vi "Add Frames.vi"(8 "error in (no error)":errorcluster, 11 "Node Ptr":u64 format="%.0x") -> ()   [LabVIEW 2020, in "FlexRay Custom Device System Explorer.lvlib"]
uses:
  FlexRay Custom Device System Explorer.lvlib
  Shared/FRConfig.ctl
  Shared/FRInterface.ctl
  <vilib>/Utility/error.llb/DialogType.ctl
  Shared/AddFramesState.ctl
  Shared/FRFrameType.ctl
  <vilib>/NI VeriStand/Custom Device API/Custom Device Channel Type.ctl
  <vilib>/NI VeriStand/Custom Device API/Custom Device Item Ref.ctl
  <vilib>/NI VeriStand/Custom Device API/Custom Device Channel.ctl
  Shared/Constants.vi
  <vilib>/NI VeriStand/Custom Device API/Get Item Property (Variant).vi
  Shared/FlexRay Custom Device Shared.lvlib
  <resource>/objmgr/xnet.rc
  <vilib>/NI VeriStand/Custom Device API/Custom Device API.lvlib
panel:
  in  "Add Selection":bool
  in  "Frames":i32[](listbox)
  in  "Reverse":bool
  in  "Cancel":bool
  in  "Add All":bool
  in  "ECU":u16(ring)
  out "error out":errorcluster
  in  "Tag":string
  # "Use ctrl or shift to select multiple frames"
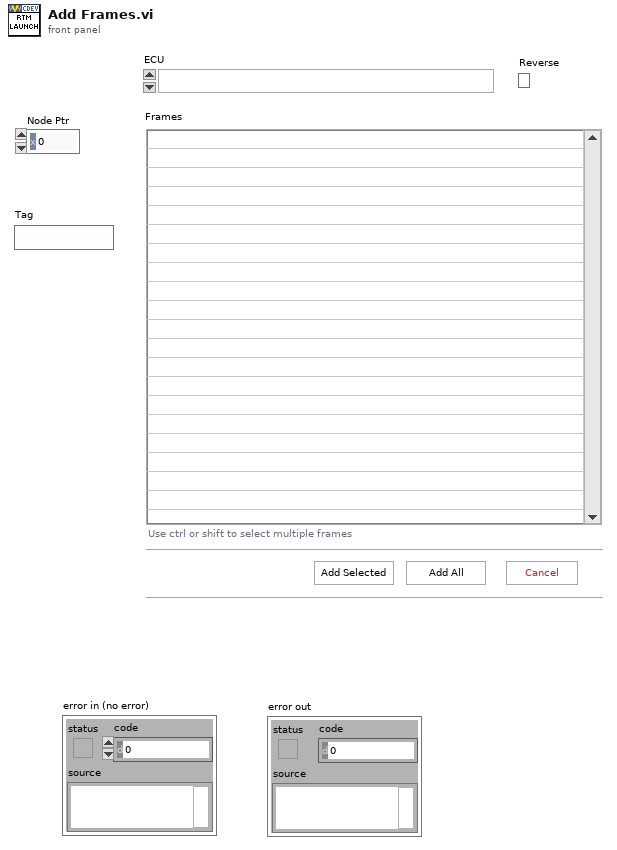
[diagram p1: front panel]
types:
  T1 = typedef "FlexRay Custom Device Shared.lvlib/AddFramesState.ctl" = enum16{"Init", "UserInput", "Action", "Cleanup"}
  T2 = typedef "DialogType.ctl" = u16
  T3 = typedef "FlexRay Custom Device Shared.lvlib/FRConfig.ctl" = cluster{"FlexRay Interface":T4, "XNET Database":refnum<k21>, "XNET Cluster":refnum<k21>, "ColdStart ID":u32, "Termination":bool}
  T4 = typedef "FlexRay Custom Device Shared.lvlib/FRInterface.ctl" = u16
  T5 = typedef "Custom Device API.lvlib/Custom Device Item Info.ctl" = cluster{"Name":string, "Is Channel":bool, "GUID":string, "Is Waveform":bool}
  T6 = typedef "Custom Device API.lvlib/Custom Device Item Ref.ctl" = u64
  T7 = typedef "Custom Device API.lvlib/Custom Device Channel Type.ctl" = enum16{"Input", "Output"}
  T8 = typedef "FlexRay Custom Device Shared.lvlib/FRFrameType.ctl" = u32
  T9 = typedef "Custom Device API.lvlib/Custom Device Channel.ctl" = cluster{"Type":T7, "Units":string, "Default Value":dbl, "Faultable":bool, "Scalable":bool}
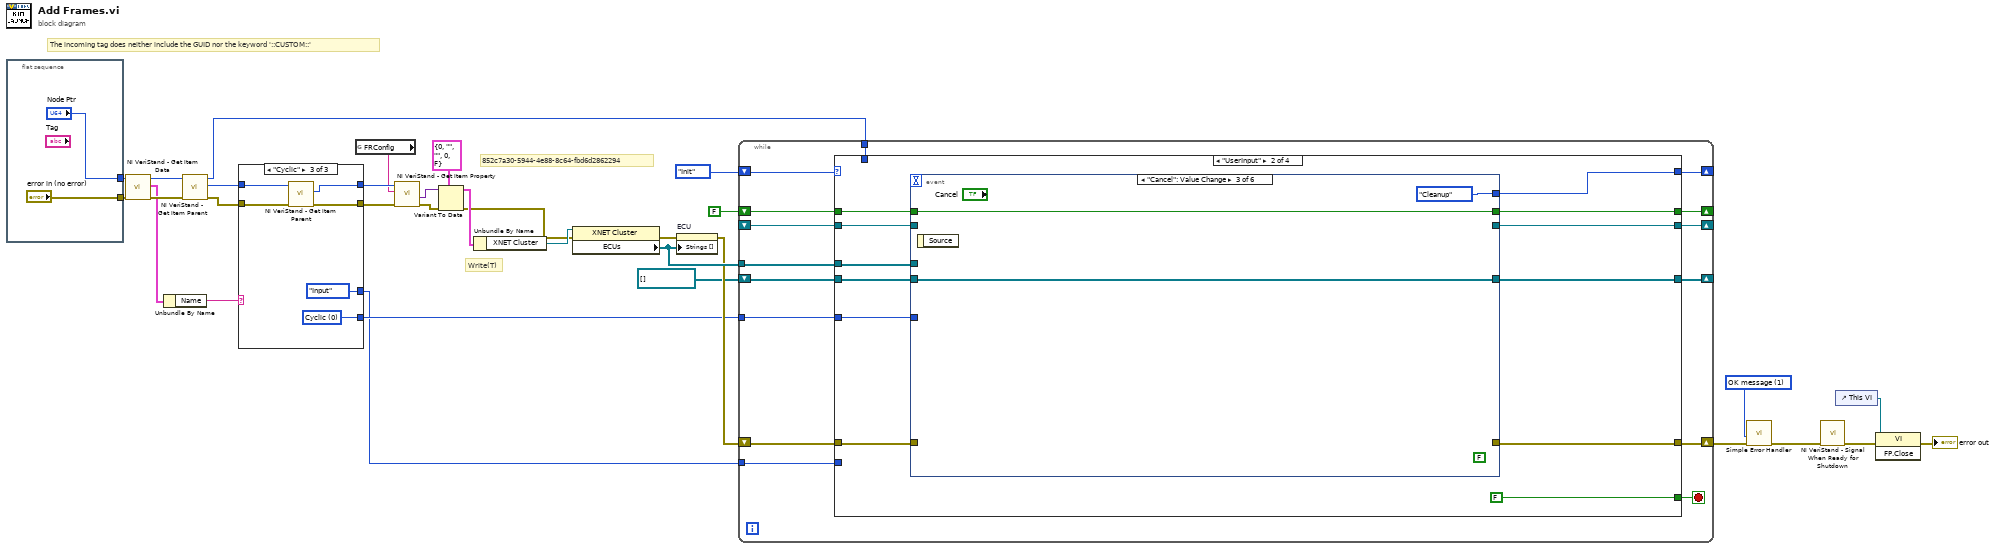
[diagram p0: block diagram]
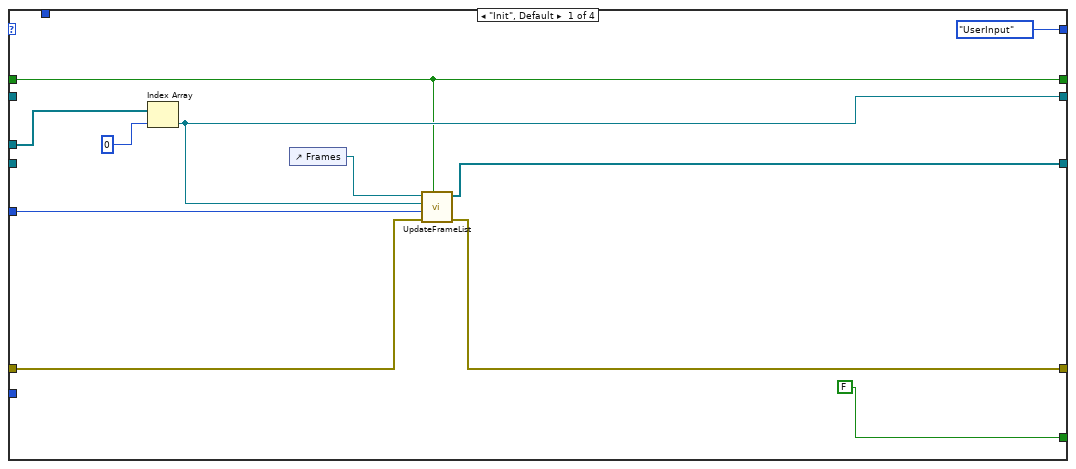
[diagram p2: hidden frame]
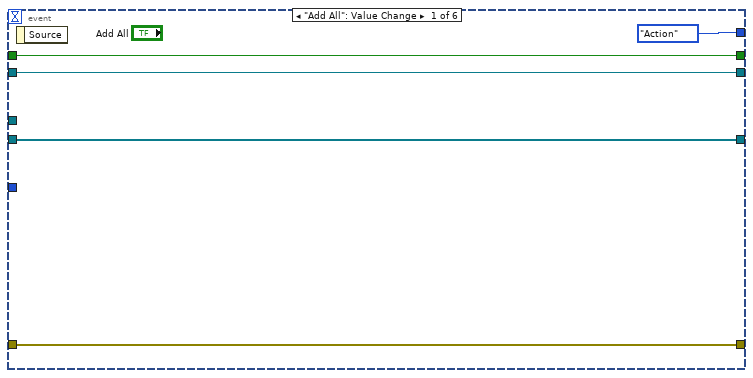
[diagram p3: hidden frame]
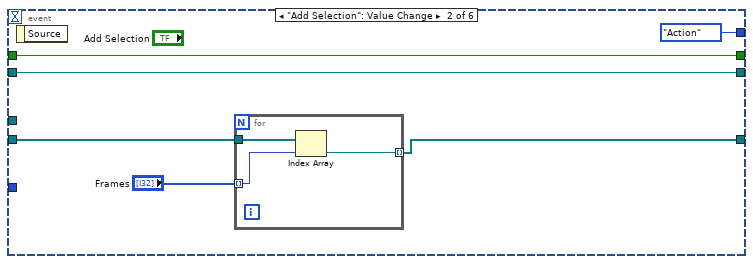
[diagram p4: hidden frame]
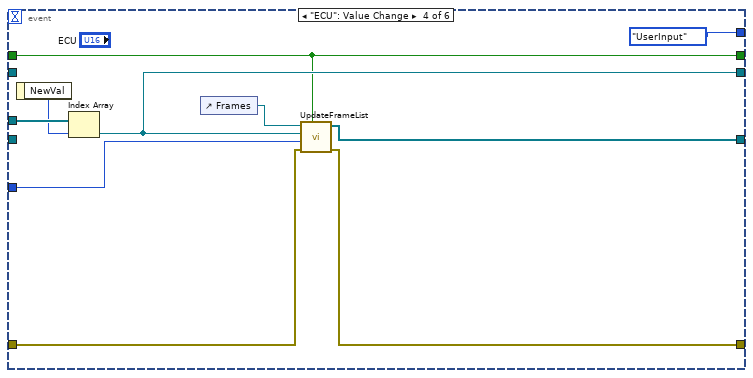
[diagram p5: hidden frame]
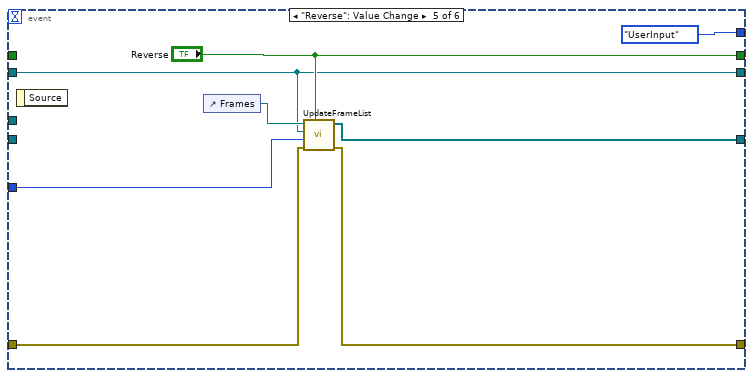
[diagram p6: hidden frame]
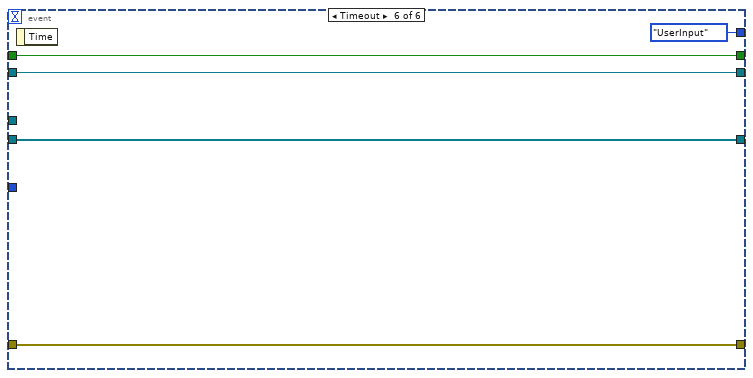
[diagram p7: hidden frame]
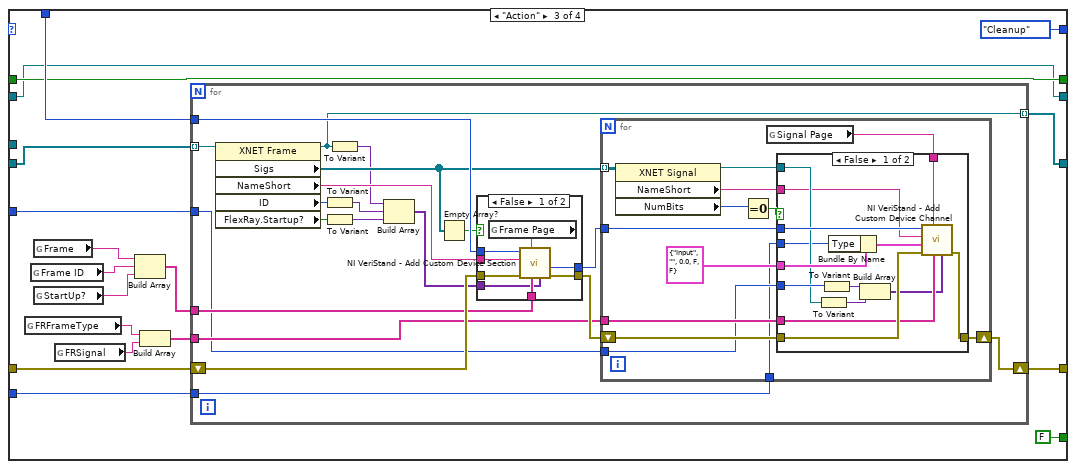
[diagram p8: hidden frame]
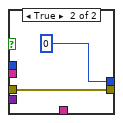
[diagram p9: hidden frame]
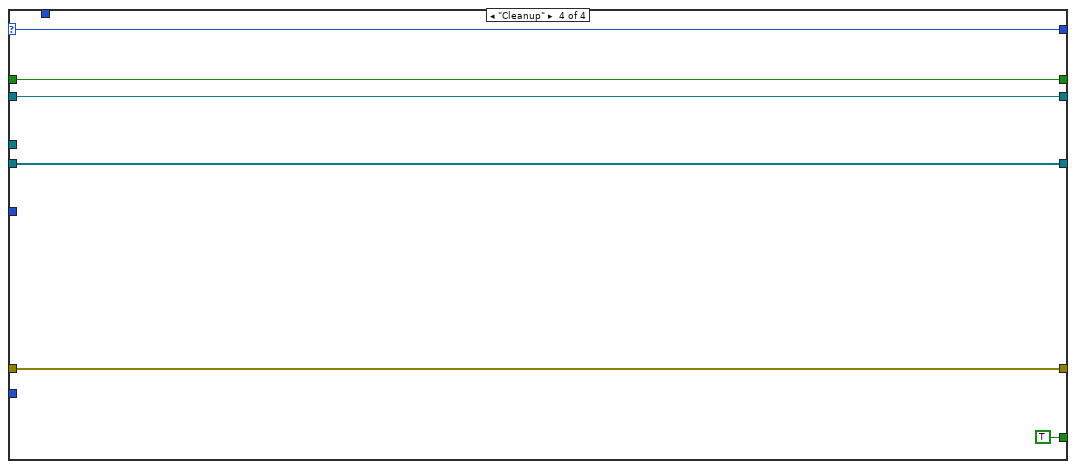
[diagram p11: hidden frame]
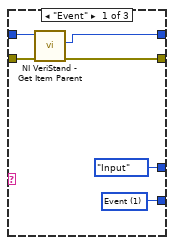
[diagram p12: hidden frame]
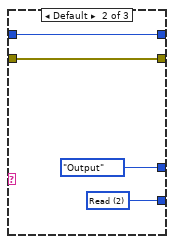
[diagram p13: hidden frame]
diagram:
  w12 = T2 1 items=["no dialog", "OK message", "continue or stop message", "OK message + warnings", "continue/stop + warnings"] ("type of dialog (OK msg:1)")
  # "852c7a30-5944-4e88-8c64-fbd6d2862294"
  # "Write(T)"
  # "The incoming tag does neither include the GUID nor the keyword '::CUSTOM::'"
  n1 = flat-sequence {
    tunnel: ["Node Ptr"] -> w24
    tunnel: ["error in (no error)"] -> w23
    frame #0 {
    }
  }
  n2 = call <vilib>:"NI VeriStand - Get Item Data.vi"("error in (no error)"=w23, "Item Ref in"=w24) -> ("error out"=w22:errorcluster, "Item Info"=w21:T5, "Item Ref out"=w5:T6)  [unwired: 6 in, 1 out]
  n3 = Unbundle By Name(w21) -> ("Name"=w20:string)
  n4 = call <vilib>:"NI VeriStand - Get Item Parent.vi"("error in (no error)"=w22, "Item Ref in"=w5) -> ("error out"=w14:errorcluster, "Parent Ref"=w26:T6, "Item Ref out"=w1:T6)  [unwired: 6 in, 1 out]
  n5 = case shown="\"Cyclic\"" w20 {
    tunnel: [w36 w42 w50] -> w4
    tunnel: w26 -> [w40 w44 w49]
    tunnel: [w39 w44 w48] -> w19
    tunnel: w14 -> [w38 w43 w47]
    tunnel: [w37 w43 w46] -> w25
    tunnel: [Custom_Device_Channel_Type."Input" ("Type") Custom_Device_Channel_Type."Output" ("Type") Custom_Device_Channel_Type."Input" ("Type")] -> w2
    frame "Event" {
      w36 = T8 1 items=["Cyclic", "Event", "Read"] ("FlexRay:Timing Type")
      n6 = call <vilib>:"NI VeriStand - Get Item Parent.vi"("error in (no error)"=w38, "Item Ref in"=w40) -> ("error out"=w37:errorcluster, "Parent Ref"=w39:T6)  [unwired: 6 in, 2 out]
    }
    frame Default {
      w42 = T8 2 items=["Cyclic", "Event", "Read"] ("FlexRay:Timing Type")
    }
    frame "Cyclic" {
      w50 = T8 0 items=["Cyclic", "Event", "Read"] ("FlexRay:Timing Type")
      n7 = call <vilib>:"NI VeriStand - Get Item Parent.vi"("error in (no error)"=w47, "Item Ref in"=w49) -> ("error out"=w46:errorcluster, "Parent Ref"=w48:T6)  [unwired: 6 in, 2 out]
    }
  }
  n8 = global read "Constants.vi" "FRConfig"() -> (w18:string)
  n9 = call-poly <vilib>:"NI VeriStand - Get Item Property.vi"("error in (no error)"=w25, "Property Name"=w18, "Item Ref in"=w19) -> ("error out"=w31:errorcluster, "Value"=w32:variant)  [unwired: 5 in, 2 out]
  n10 = Variant To Data(error in=w31, type=T3 {"FlexRay Interface"=0, "XNET Database"="", "XNET Cluster"="", "ColdStart ID"=0, "Termination"=FALSE} ("FRConfig"), Variant=w32) -> (data=w29:T3, error out=w27:errorcluster)
  n11 = Unbundle By Name(w29) -> ("XNET Cluster"=w28:refnum<k21>)
  n12 = property class="XNET Cluster"(reference=w28, error in=w27) -> (error out=w10:errorcluster, "ECUs"=w11:refnum<k21>[])  [unwired: 1 out]
  n13 = property on="ECU" class="Ring (strict)"(error in=w10, "Strings []"=w11) -> (error out=w9:errorcluster)  [unwired: 1 in, 1 out]
  n14 = while {
    tunnel: w11 -> [w65]
    tunnel: w4 -> [w63]
    shift-right: [w52] -> _
    shift-left: refnum<k21>[] [] -> [w62]
    shift-right: [w53] -> w3
    shift-left: w9 -> [w61]
    shift-right: [w60] -> _
    shift-left: FALSE ("Reverse") -> [w59]
    shift-right: [w55] -> _
    shift-left: AddFramesState."Init" -> [w57]
    shift-right: [w58] -> _
    shift-left: _ -> [w56]
    tunnel: w1 -> [w54]
    tunnel: w2 -> [w51]
    stop <- w64 stop-if-true
    n15 = case shown="\"UserInput\"" w57 {
      selector: w57 -> [_ _ _ w210]
      tunnel: w65 -> [w76 w88 _ _]
      tunnel: [FALSE FALSE FALSE TRUE] -> w64
      tunnel: w63 -> [w72 w87 w130 _]
      tunnel: [w66 w86 w132 w207] -> w52
      tunnel: w62 -> [_ w85 w134 w207]
      tunnel: [w68 w84 w138 w208] -> w53
      tunnel: w61 -> [w70 w83 w133 w208]
      tunnel: [w69 w82 w137 w205] -> w60
      tunnel: w59 -> [w69 w81 w137 w205]
      tunnel: [w71 w80 w136 w206] -> w58
      tunnel: w56 -> [_ w77 w136 w206]
      tunnel: [AddFramesState."UserInput" w79 AddFramesState."Cleanup" w210] -> w55
      tunnel: w54 -> [_ _ w139 _]
      tunnel: w51 -> [_ _ w129 _]
      frame "Init", Default {
        n16 = Index Array(array=w76, index=0) -> (element=w71:refnum<k21>)
        n17 = control-ref of="Frames"() -> (w67:refnum<vi>)
        n18 = call "UpdateFrameList.vi"("Reverse"=w69, "error in (no error)"=w70, "FlexRay:Timing Type"=w72, "XNET ECU"=w71, "ListBox in"=w67) -> ("error out"=w68:errorcluster, "Frames"=w66:refnum<k21>[])  [unwired: 5 in]
      }
      frame "UserInput" {
        n19 = event shown="[2] \"Cancel\": Value Change" {
          selector: _ -> [_ _ _ _ _ _]
          dyn-events: _ -> [_ _ _ _ _ _]
          timeout: _ -> [_ _ _ _ _ _]
          tunnel: w88 -> [_ _ _ w115 _ _]
          tunnel: w87 -> [_ _ _ w110 w119 _]
          tunnel: [w91 w94 w105 w107 w118 w127] -> w86
          tunnel: w85 -> [w91 w95 w105 _ _ w127]
          tunnel: [w89 _ _ w108 w117 w128] -> w84
          tunnel: w83 -> [w89 _ _ w109 w116 w128]
          tunnel: [w93 w98 w104 w111 "Reverse" w126] -> w82
          tunnel: w81 -> [w93 w98 w104 w111 _ w126]
          tunnel: [w90 w97 _ w112 w120 w125] -> w80
          tunnel: [AddFramesState."Action" AddFramesState."Action" AddFramesState."Cleanup" AddFramesState."UserInput" AddFramesState."UserInput" AddFramesState."UserInput"] -> w79
          tunnel: w77 -> [w90 w97 _ _ w120 w125]
          event "Add All": Value Change {
            n20 = event-data() -> ()  [unwired: 1 in, 1 out]
          }
          event "Add Selection": Value Change {
            n21 = event-data() -> ()  [unwired: 1 in, 1 out]
            n22 = for {
              tunnel: "Frames" -> [w101] mode=indexing
              tunnel: w95 -> [w102]
              tunnel: [w100] -> w94 mode=indexing
              n23 = Index Array(array=w102, index=w101) -> (element=w100:refnum<k21>)
            }
          }
          event "Cancel": Value Change {
            (unwired) FALSE
            n24 = event-data() -> ()  [unwired: 1 in, 1 out]
          }
          event "ECU": Value Change {
            n25 = event-data() -> ("NewVal"=w114:u16)  [unwired: 1 in]
            n26 = Index Array(array=w115, index=w114) -> (element=w112:refnum<k21>)
            n27 = control-ref of="Frames"() -> (w106:refnum<vi>)
            n28 = call "UpdateFrameList.vi"("Reverse"=w111, "error in (no error)"=w109, "FlexRay:Timing Type"=w110, "XNET ECU"=w112, "ListBox in"=w106) -> ("error out"=w108:errorcluster, "Frames"=w107:refnum<k21>[])  [unwired: 5 in]
          }
          event "Reverse": Value Change {
            n29 = event-data() -> ()  [unwired: 1 in, 1 out]
            n30 = control-ref of="Frames"() -> (w122:refnum<vi>)
            n31 = call "UpdateFrameList.vi"("Reverse"="Reverse", "error in (no error)"=w116, "FlexRay:Timing Type"=w119, "XNET ECU"=w120, "ListBox in"=w122) -> ("error out"=w117:errorcluster, "Frames"=w118:refnum<k21>[])  [unwired: 5 in]
          }
          event Timeout {
            n32 = event-data() -> ()  [unwired: 1 in, 1 out]
          }
        }
      }
      frame "Action" {
        n33 = global read "Constants.vi" "FRFrameType"() -> (w141:string)
        n34 = global read "Constants.vi" "Frame ID"() -> (w143:string)
        n35 = global read "Constants.vi" "Frame"() -> (w146:string)
        n36 = global read "Constants.vi" "StartUp?"() -> (w144:string)
        n37 = global read "Constants.vi" "FRSignal"() -> (w140:string)
        n38 = Build Array(w146, w143, w144) -> (w145:string[])
        n39 = Build Array(w141, w140) -> (w142:string[])
        n40 = for {
          shift-right: [w160] -> w138
          shift-left: w133 -> [w163]
          tunnel: w134 -> [w166] mode=indexing
          tunnel: w139 -> [w165]
          tunnel: w142 -> [w159]
          tunnel: w145 -> [w158]
          tunnel: [w149] -> w132 mode=indexing
          tunnel: w130 -> [w148]
          tunnel: w129 -> [w147]
          n41 = property class="XNET Frame"(reference=w166) -> (reference out=w149:refnum<k21>, "Sigs"=w151:refnum<k21>[], "NameShort"=w164:string, "ID"=w157:u32, "FlexRay.Startup?"=w156:bool)  [unwired: 1 in, 1 out]
          n42 = To Variant(anything=w157) -> (Variant=w155:variant)
          n43 = To Variant(anything=w156) -> (Variant=w154:variant)
          n44 = To Variant(anything=w149) -> (Variant=w150:variant)
          n45 = Build Array(w150, w155, w154) -> (w153:variant[])
          n46 = Empty Array?(array=w151) -> (empty?=w152:bool)
          n47 = case shown="False" w152 {
            tunnel: w165 -> [w174 _]
            tunnel: w164 -> [w173 _]
            tunnel: w163 -> [w171 w176]
            tunnel: [w170 T6 0 ("Section Ptr")] -> w162
            tunnel: [w169 w176] -> w161
            tunnel: w158 -> [w168 _]
            tunnel: w153 -> [w167 _]
            frame False {
              n48 = global read "Constants.vi" "Frame Page"() -> (w172:string)
              n49 = call <vilib>:"NI VeriStand - Add Custom Device Section.vi"("Property Values"=w167, "Property names"=w168, "GUID (Default Section)"=w172, "error in (no error)"=w171, "Section Name"=w173, "Parent Ref in"=w174) -> ("error out"=w169:errorcluster, "Section Ptr"=w170:T6)  [unwired: 2 in, 2 out]
            }
            frame True {
            }
          }
          n50 = for {
            tunnel: w151 -> [w183] mode=indexing
            tunnel: w162 -> [w189]
            shift-right: [w186] -> w160
            shift-left: w161 -> [w187]
            tunnel: w159 -> [w184]
            tunnel: w148 -> [w178]
            tunnel: w147 -> [w177]
            n51 = property class="XNET Signal"(reference=w183) -> (reference out=w182:refnum<k21>, "NameShort"=w181:string, "NumBits"=w179:u32)  [unwired: 1 in, 1 out]
            n52 = Equal To 0?(x=w179) -> (x = 0?=w180:bool)
            n53 = global read "Constants.vi" "Signal Page"() -> (w185:string)
            n54 = case shown="False" w180 {
              tunnel: w189 -> [w203 _]
              tunnel: T9 {"Type"=enum."Input", "Units"="", "Default Value"=0.0, "Faultable"=FALSE, "Scalable"=FALSE} ("Channel") -> [w202 _]
              tunnel: w187 -> [w200 w204]
              tunnel: [w199 w204] -> w186
              tunnel: w185 -> [w198 _]
              tunnel: w184 -> [w197 _]
              tunnel: w178 -> [w193 _]
              tunnel: w182 -> [w192 _]
              tunnel: w181 -> [w191 _]
              tunnel: w177 -> [w190 _]
              frame False {
                n55 = To Variant(anything=w192) -> (Variant=w195:variant)
                n56 = To Variant(anything=w193) -> (Variant=w196:variant)
                n57 = Bundle By Name(cluster=w202, "Type"=w190) -> (w201:T9)
                n58 = Build Array(w196, w195) -> (w194:variant[])
                n59 = call <vilib>:"NI VeriStand - Add Custom Device Channel.vi"("Property Values"=w194, "Property names"=w197, "GUID (Default Channel)"=w198, "error in (no error)"=w200, "Channel"=w201, "Channel Name"=w191, "Parent Ref in"=w203) -> ("error out"=w199:errorcluster)  [unwired: 1 in, 3 out]
              }
              frame True {
              }
            }
          }
        }
      }
      frame "Cleanup" {
      }
    }
  }
  n60 = call <vilib>:"Simple Error Handler.vi"("type of dialog (OK msg:1)"=w12, "error in (no error)"=w3) -> ("error out"=w13:errorcluster)  [unwired: 3 in, 4 out]
  n61 = call <vilib>:"NI VeriStand - Signal When Ready for Shutdown.vi"("error in (no error)"=w13) -> ("error out"=w17:errorcluster)  [unwired: 10 in]
  n62 = control-ref of="This VI"() -> (w15:refnum<vi>)
  n63 = invoke class="VI" method="FP.Close"(reference=w15, error in=w17) -> (error out=→"error out":errorcluster)  [unwired: 1 in, 2 out]
